vi "Push button and turn on LED.vi"() -> ()   [LabVIEW 2010]
doc: "This example shows how to control Red Pitaya on board LEDs and read states of extension connector GPIOs.\nLED will turn ON, when button is pressed."
uses:
  RedPitaya.lvlib
panel:
  in  "LED ON when":u16(ring) items=["High"=1, "Low"=0]
  in  "LED #":u16(ring)=5 items=["LED1"=1, "LED2"=2, "LED3"=3, "LED4"=4, "LED5"=5, "LED6"=6, "LED7"=7]
  in  "Pin #":string="DIO5_N"
  in  "stop":bool
  in  "IP address":string="192.168.4.129"
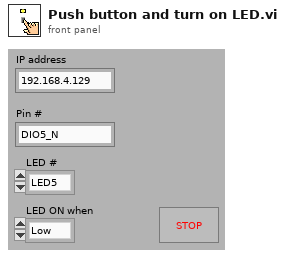
[diagram p1: front panel]
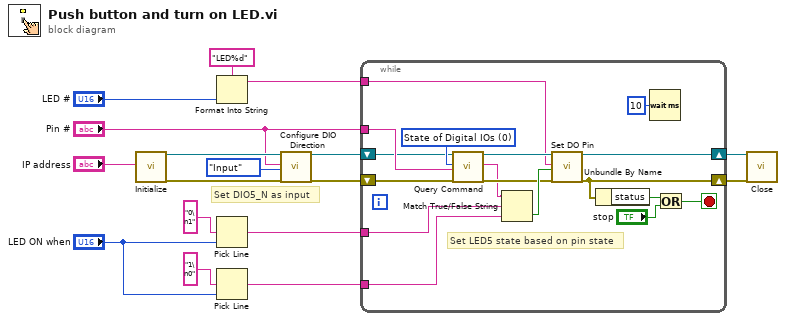
[diagram p0: block diagram]
diagram:
  # "Set DIO5_N as input"
  n1 = call "Initialize.vi"("IP address"="IP address") -> ("RedPitaya connection out"=w16:refnum<k5>, "error out"=w15:errorcluster)  [unwired: 17 in]
  n2 = Format Into String(format string="LED%d", "LED #") -> (resulting string=w7:string)  [unwired: 2 in, 1 out]
  n3 = Pick Line(multi-line string="0\n1" ("true string"), line index="LED ON when") -> (output string=w3:string)  [unwired: 1 in]
  n4 = Pick Line(multi-line string="1\n0" ("false string"), line index="LED ON when") -> (output string=w2:string)  [unwired: 1 in]
  n5 = call "Configure DIO Direction.vi"("RedPitaya connection in"=w16, "Pin name"="Pin #", "Direction"=enum16{"Output", "Input"}."Input", "error in"=w15) -> ("RedPitaya connection out"=w14:refnum<k5>, "error out"=w13:errorcluster)  [unwired: 14 in]
  n6 = while {
    tunnel: "Pin #" -> [w33]
    shift-right: [w27] -> w12
    shift-left: w14 -> [w31]
    shift-right: [w21] -> w11
    shift-left: w13 -> [w30]
    tunnel: w7 -> [w24]
    tunnel: w3 -> [w23]
    tunnel: w2 -> [w22]
    stop <- w20 stop-if-true
    w34 = u16 0 items=["State of Digital IOs", "Analog Voltage", "Decimation", "Sampling Rate", "Sampling Rate (Hz)", "Averaging Status", "Trigger Status", "Trigger Delay in Samples", "Trigger Delay in Nanoseconds", "Trigger Level in mV", "Current Position of Write Pointer", "Position of Trigger Event", "Buffer Size"] ("Query setting")
    # "Set LED5 state based on pin state"
    n7 = call "Query Command.vi"("RedPitaya connection in"=w31, "Query setting"=w34, "Pin Name"=w33, "error in"=w30) -> ("RedPitaya connection out"=w29:refnum<k5>, "Output string"=w25:string, "error out"=w28:errorcluster)  [unwired: 13 in]
    n8 = Match True/False String(2:w22, 3:w23, 4:w25) -> (0:w32:bool)  [unwired: 1 out]
    n9 = call "Set DO Pin.vi"("RedPitaya connection in"=w29, "Pin name"=w24, "State"=w32, "error in"=w28) -> ("RedPitaya connection out"=w27:refnum<k5>, "error out"=w21:errorcluster)  [unwired: 14 in]
    n10 = Unbundle By Name(w21) -> ("status"=w19:bool)
    n11 = Wait (ms)(milliseconds to wait=u32 10) -> ()  [unwired: 1 out]
    n12 = Or(x=w19, y="stop") -> (x .or. y?=w20:bool)
  }
  n13 = call "Close.vi"("RedPitaya connection in"=w12, "error in"=w11) -> ()  [unwired: 17 in, 1 out]
